vi "New DynamicPersonality.vi"(6 "Pinned":T9={"Attacker"="None", "Striker"="None", "Defender"="None", "Goalie"="None"}, 9 "Maior prioridade de \natacante é o mais\nproximo da bola?":bool, 10 "our_goalie_id":dbl, 11 "input cluster":T1) -> (2 "output cluster":T1)   [LabVIEW 2016]
uses:
  Util/Select Auto None or Robot.ctl
  Core/AI Input.ctl
  Core/AI Robot.ctl
  Intel/Functions Enum.ctl
  Core/AI Ball.ctl
  Core/Field Size.ctl
  Core/AI Judge.ctl
  Intel/Command Enum.ctl
panel:
  out "Strk\nPinned?":bool
  out "Attck\nPinned?":bool
  in  "Ids validos":u32[](array[numeric])=[42, 42, 42, 42, 42, 42, 42]
  in  "Total de Robôs":dbl format="%#_13g"
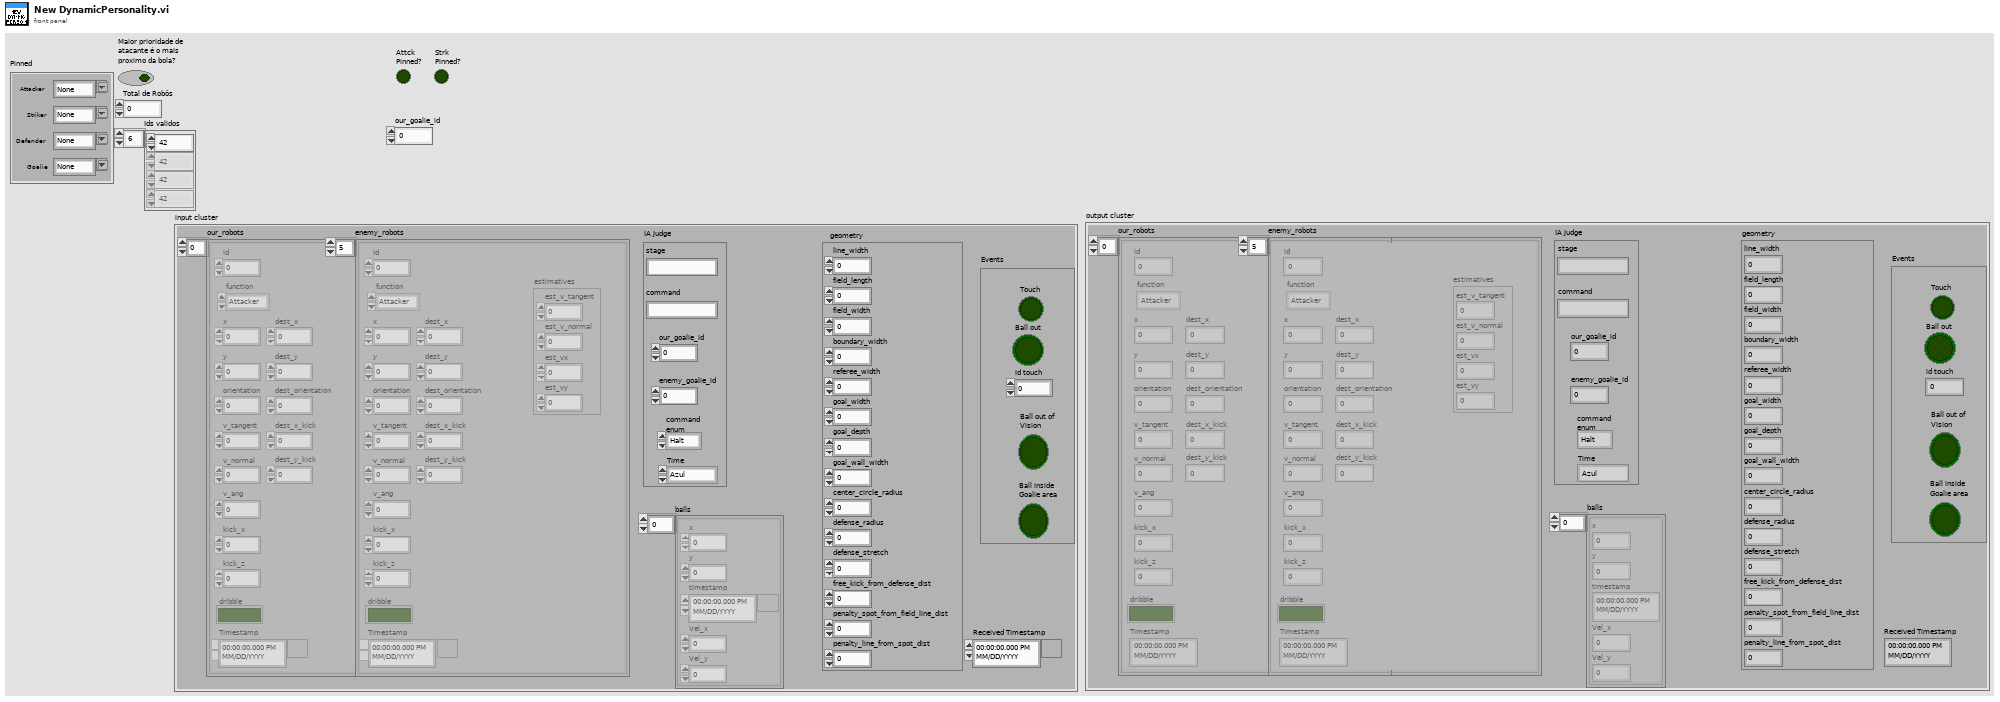
[diagram p1: front panel]
types:
  T1 = typedef "AI Input.ctl" = cluster{"our_robots":T2[], "enemy_robots":T2[], "balls":T4[], "geometry":T5, "IA Judge":T6, "Received Timestamp":timestamp, "Events":cluster{"Touch":bool, "Ball out":bool, "id touch":dbl, "Ball out of \nVision":bool, "Ball inside \nGoalie area":bool}}
  T2 = typedef "AI Robot.ctl" = cluster{"id":u32, "function":T3, "x":dbl, "y":dbl, "orientation":dbl, "v_tangent":dbl, "v_normal":dbl, "v_ang":dbl, "kick_x":dbl, "kick_z":dbl, "dribble":bool, "Timestamp":timestamp, "dest_x":dbl, "dest_y":dbl, "dest_orientation":dbl, "estimatives":cluster{"est_v_tangent":dbl, "est_v_normal":dbl, "est_vx":dbl, "est_vy":dbl}, "dest_x_kick":dbl, "dest_y_kick":dbl}
  T3 = typedef "Functions Enum.ctl" = enum16{"Attacker", "Goalie", "Defender", "Striker", "Goto 0", "Dummy", "ZigZag"}
  T4 = typedef "AI Ball.ctl" = cluster{"x":dbl, "y":dbl, "timestamp":timestamp, "Vel_x":dbl, "Vel_y":dbl}
  T5 = typedef "Field Size.ctl" = cluster{"line_width":u32, "field_length":u32, "field_width":u32, "boundary_width":u32, "referee_width":u32, "goal_width":u32, "goal_depth":u32, "goal_wall_width":u32, "center_circle_radius":u32, "defense_radius":u32, "defense_stretch":u32, "free_kick_from_defense_dist":u32, "penalty_spot_from_field_line_dist":u32, "penalty_line_from_spot_dist":u32}
  T6 = typedef "AI Judge.ctl" = cluster{"stage":string, "command":string, "our_goalie_id":dbl, "enemy_goalie_id":dbl, "command\nenum":T7, "Time":enum16{"Azul", "Amarelo"}}
  T7 = typedef "Command Enum.ctl" = enum16{"Halt", "Stop", "Force Start", "PKA Normal Start", "Prepare Kickoff Ally", "PKE Normal Start", "Prepare Kickoff Enemy", "Prepare Penalty Ally", "PPA Normal Start", "Prepare Penalty Enemy", "PPE Normal Start", "Direct Free Enemy", "Direct Free Ally", "Indirect Free Enemy", "Indirect Free Ally", "Timeout Enemy", "Timeout Ally", "Goal Enemy", "Goal Ally", "Ball Placement Enemy", "Ball Placement Ally", "None"}
  T8 = typedef "Select Auto None or Robot.ctl" = string
  T9 = cluster{"Attacker":T8, "Striker":T8, "Defender":T8, "Goalie":T8}
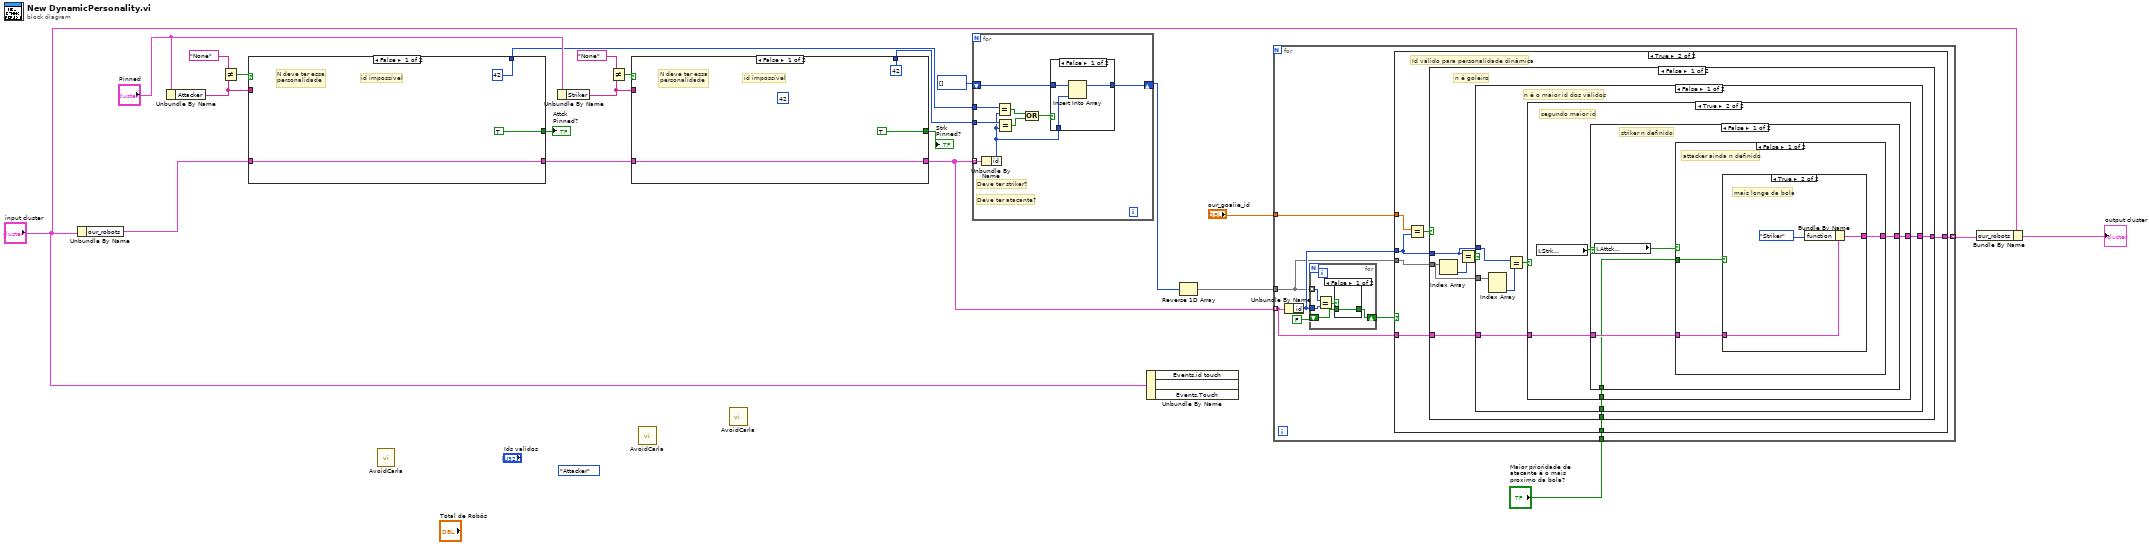
[diagram p0: block diagram]
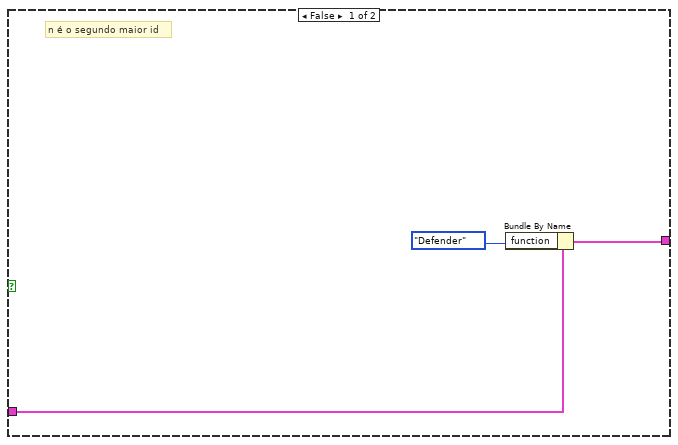
[diagram p3: hidden frame]
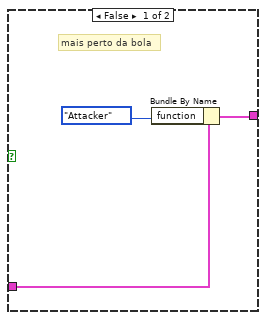
[diagram p4: hidden frame]
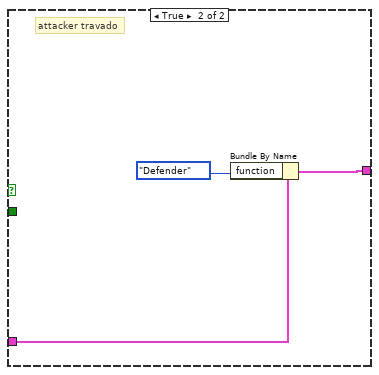
[diagram p5: hidden frame]
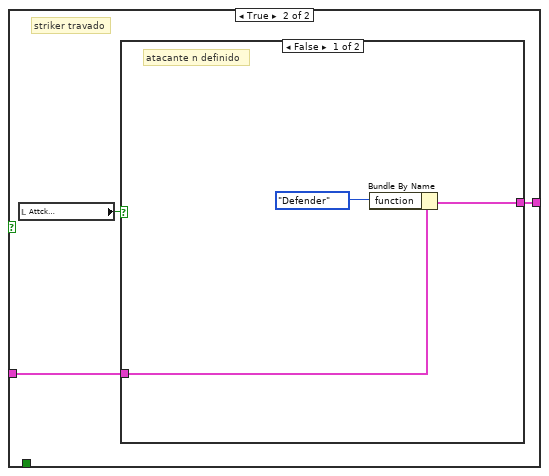
[diagram p6: hidden frame]
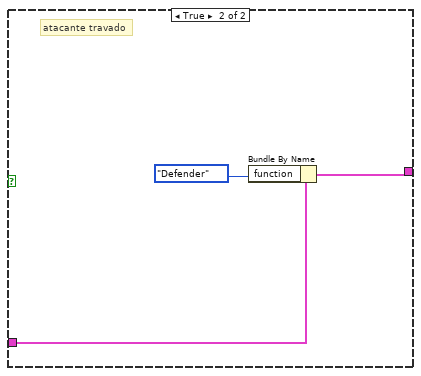
[diagram p7: hidden frame]
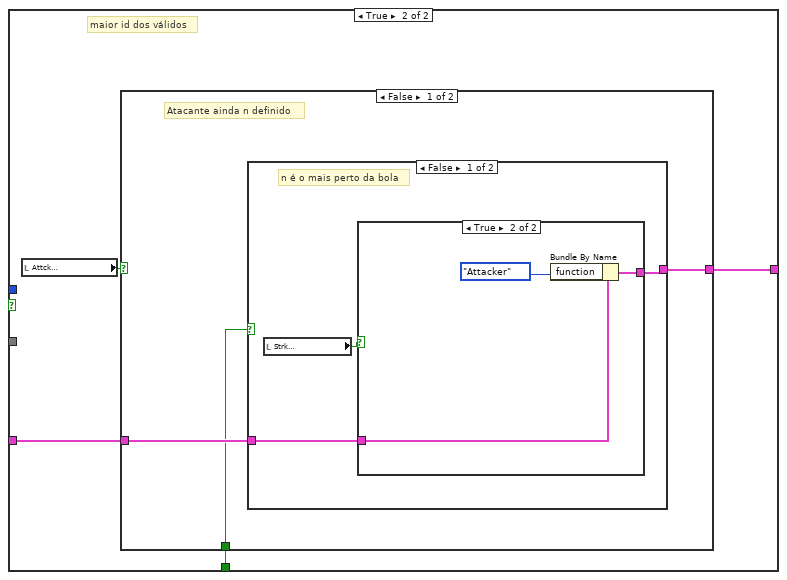
[diagram p8: hidden frame]
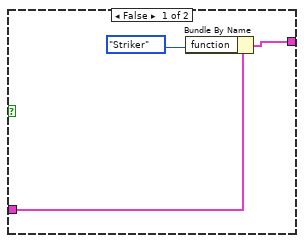
[diagram p9: hidden frame]
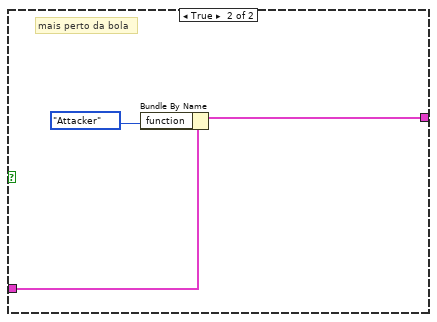
[diagram p10: hidden frame]
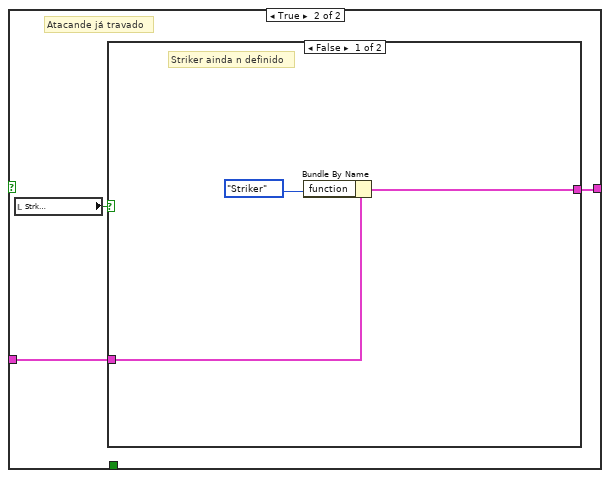
[diagram p11: hidden frame]
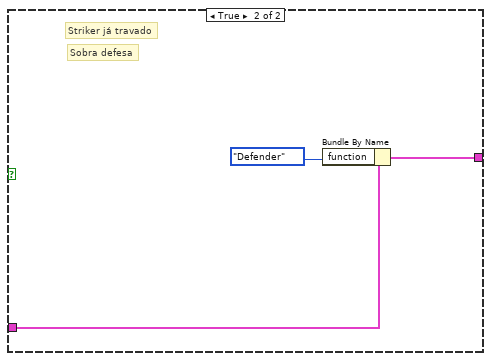
[diagram p12: hidden frame]
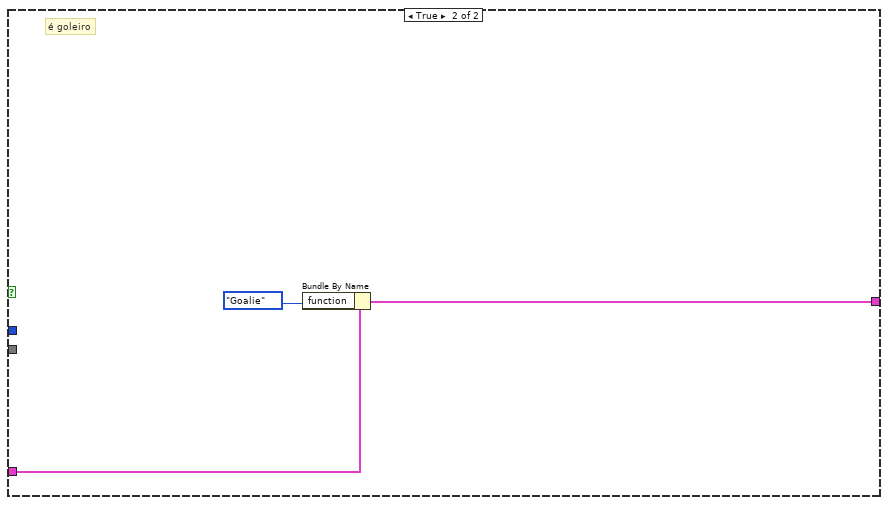
[diagram p13: hidden frame]
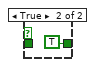
[diagram p14: hidden frame]
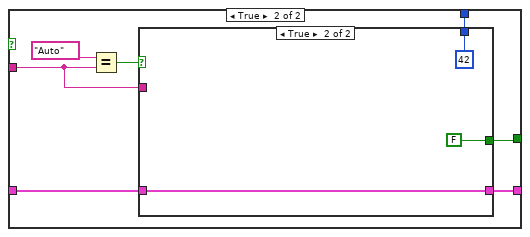
[diagram p16: hidden frame]
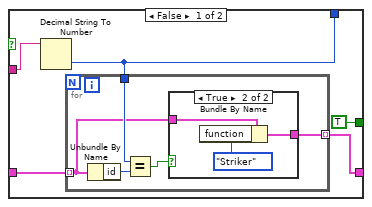
[diagram p17: hidden frame]
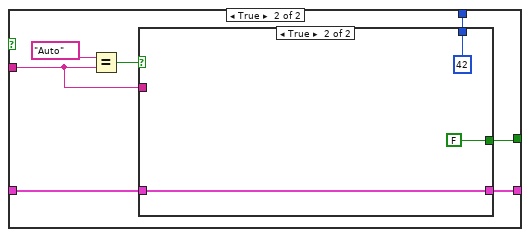
[diagram p19: hidden frame]
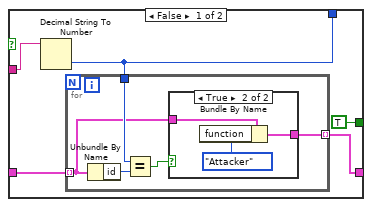
[diagram p20: hidden frame]
diagram:
  (unwired) Functions_Enum."Attacker" ("function")
  n1 = Unbundle By Name("input cluster") -> ("our_robots"=w19:T2[])
  n2 = Unbundle By Name("Pinned") -> ("Attacker"=w20:T8)
  n3 = Not Equal?(x=T8 "None", y=w20) -> (x != y?=w21:bool)
  n4 = case shown="False" w21 {
    tunnel: w20 -> [_ w30]
    tunnel: w19 -> [w25 w29]
    tunnel: [w25 w28] -> w15
    tunnel: [TRUE w27] -> w6
    tunnel: [u32 42 ("Id Maior\nprioridade\natacante") w26] -> w12
    frame False {
      # "id impossível"
      # "N deve ter essa \npersonalidade"
    }
    frame True {
      n5 = Equal?(x=T8 "Auto", y=w30) -> (x = y?=w31:bool)
      n6 = case shown="True" w31 {
        tunnel: w30 -> [w37 _]
        tunnel: w29 -> [w36 w49]
        tunnel: [w35 w49] -> w28
        tunnel: [TRUE FALSE] -> w27
        tunnel: [w33 42] -> w26
        frame False {
          n7 = Decimal String To Number(string=w37) -> (number=w33:i32)  [unwired: 2 in, 1 out]
          n8 = for {
            tunnel: w36 -> [w40] mode=indexing
            tunnel: w33 -> [w41]
            tunnel: [w39] -> w35 mode=indexing
            n9 = Unbundle By Name(w40) -> ("id"=w42:u32)
            n10 = Equal?(x=w41, y=w42) -> (x = y?=w38:bool)
            n11 = case shown="True" w38 {
              tunnel: w40 -> [w43 w46]
              tunnel: [w43 w45] -> w39
              frame False {
              }
              frame True {
                n12 = Bundle By Name(cluster=w46, "function"=Functions_Enum."Attacker") -> (w45:T2)
              }
            }
          }
        }
        frame True {
        }
      }
    }
  }
  "Attck\nPinned?" <- w6
  n13 = call "AvoidCarla.vi"() -> ()  [unwired: 11 in, 1 out]
  n14 = Unbundle By Name("Pinned") -> ("Striker"=w17:T8)
  n15 = Not Equal?(x=T8 "None", y=w17) -> (x != y?=w14:bool)
  n16 = case shown="False" w14 {
    tunnel: w17 -> [_ w57]
    tunnel: w15 -> [w52 w56]
    tunnel: [w52 w55] -> w10
    tunnel: [TRUE w54] -> w5
    tunnel: [42 w53] -> w13
    frame False {
      (unwired) u32 42 ("Id Maior\nprioridade\natacante")
      # "id impossível"
      # "N deve ter essa \npersonalidade"
    }
    frame True {
      n17 = Equal?(x=T8 "Auto", y=w57) -> (x = y?=w58:bool)
      n18 = case shown="True" w58 {
        tunnel: w57 -> [w64 _]
        tunnel: w56 -> [w63 w76]
        tunnel: [w62 w76] -> w55
        tunnel: [TRUE FALSE] -> w54
        tunnel: [w60 42] -> w53
        frame False {
          n19 = Decimal String To Number(string=w64) -> (number=w60:i32)  [unwired: 2 in, 1 out]
          n20 = for {
            tunnel: w63 -> [w67] mode=indexing
            tunnel: w60 -> [w68]
            tunnel: [w66] -> w62 mode=indexing
            n21 = Unbundle By Name(w67) -> ("id"=w69:u32)
            n22 = Equal?(x=w68, y=w69) -> (x = y?=w65:bool)
            n23 = case shown="True" w65 {
              tunnel: w67 -> [w70 w73]
              tunnel: [w70 w72] -> w66
              frame False {
              }
              frame True {
                n24 = Bundle By Name(cluster=w73, "function"=Functions_Enum."Striker") -> (w72:T2)
              }
            }
          }
        }
        frame True {
        }
      }
    }
  }
  "Strk\nPinned?" <- w5
  n25 = call "AvoidCarla.vi"() -> ()  [unwired: 11 in, 1 out]
  n26 = call "AvoidCarla.vi"() -> ()  [unwired: 11 in, 1 out]
  n27 = for {
    tunnel: w10 -> [w85] mode=indexing
    tunnel: w13 -> [w84]
    shift-right: [w79] -> w8
    shift-left: u32[] [] -> [w80]
    tunnel: w12 -> [w83]
    # "Deve ter striker?"
    # "Deve ter atacante?"
    n28 = Unbundle By Name(w85) -> ("id"=w77:u32)
    n29 = Equal?(x=w83, y=w77) -> (x = y?=w82:bool)
    n30 = Equal?(x=w84, y=w77) -> (x = y?=w81:bool)
    n31 = Compound Arithmetic op=OR(w82, w81) -> (w78:bool)
    n32 = case shown="False" w78 {
      tunnel: [w86 w89] -> w79
      tunnel: w80 -> [w88 w89]
      tunnel: w77 -> [w87 _]
      frame False {
        n33 = Insert Into Array(array=w88, new element=w87) -> (w86:u32[])  [unwired: 1 in]
      }
      frame True {
      }
    }
  }
  n34 = Unbundle By Name("input cluster") -> ()  [unwired: 3 out]
  n35 = Reverse 1D Array(array=w8) -> (reversed array=w7:u32[])
  n36 = for {
    tunnel: w10 -> [w94] mode=indexing
    tunnel: w7 -> [w92]
    tunnel: "our_goalie_id" -> [w95]
    tunnel: [w93] -> w4 mode=indexing
    tunnel: "Maior prioridade de \natacante é o mais\nproximo da bola?" -> [w90]
    n37 = Unbundle By Name(w94) -> ("id"=w96:u32)
    n38 = for {
      tunnel: w92 -> [w186] mode=indexing
      tunnel: w96 -> [w187]
      shift-right: [w184] -> w91
      shift-left: FALSE -> [w185]
      n39 = Equal?(x=w186, y=w187) -> (x = y?=w183:bool)
      n40 = case shown="False" w183 {
        tunnel: w185 -> [w188 _]
        tunnel: [w188 TRUE] -> w184
        frame False {
        }
        frame True {
        }
      }
    }
    n41 = case shown="True" w91 {
      tunnel: w96 -> [_ w101]
      tunnel: w95 -> [_ w105]
      tunnel: w94 -> [w98 w103]
      tunnel: [w98 w102] -> w93
      tunnel: w92 -> [_ w100]
      tunnel: w90 -> [_ w99]
      frame False {
        # "Personalidade já definida"
      }
      frame True {
        # "Id válido para personalidade dinâmica"
        n42 = Equal?(x=w105, y=w101) -> (x = y?=w104:bool)
        n43 = case shown="False" w104 {
          tunnel: w103 -> [w109 w181]
          tunnel: [w110 w180] -> w102
          tunnel: w101 -> [w107 _]
          tunnel: w100 -> [w108 _]
          tunnel: w99 -> [w106 _]
          frame False {
            # "n é goleiro"
            n44 = Index Array(array=w108) -> (element=w111:u32)  [unwired: 1 in]
            n45 = Equal?(x=w107, y=w111) -> (x = y?=w112:bool)
            n46 = case shown="False" w112 {
              tunnel: [w116 w154] -> w110
              tunnel: w109 -> [w117 w153]
              tunnel: w108 -> [w118 _]
              tunnel: w107 -> [w115 _]
              tunnel: w106 -> [w113 w152]
              frame False {
                # "n é o maior id dos válidos"
                n47 = Index Array(array=w118) -> (element #2=w114:u32)  [unwired: 2 in, 1 out]
                n48 = Equal?(x=w115, y=w114) -> (x = y?=w119:bool)
                n49 = case shown="True" w119 {
                  tunnel: w117 -> [w120 w125]
                  tunnel: [w121 w124] -> w116
                  tunnel: w113 -> [_ w123]
                  frame False {
                    # "n é o segundo maior id"
                    n50 = Bundle By Name(cluster=w120, "function"=Functions_Enum."Defender") -> (w121:T2)
                  }
                  frame True {
                    # "segundo maior id"
                    n51 = local read "Strk\nPinned?"() -> (w126:bool)
                    n52 = case shown="False" w126 {
                      tunnel: w125 -> [w129 w144]
                      tunnel: [w130 w143] -> w124
                      tunnel: w123 -> [w127 _]
                      frame False {
                        # "striker n definido"
                        n53 = local read "Attck\nPinned?"() -> (w128:bool)
                        n54 = case shown="False" w128 {
                          tunnel: [w133 w141] -> w130
                          tunnel: w129 -> [w132 w140]
                          tunnel: w127 -> [w131 _]
                          frame False {
                            # "attacker ainda n definido"
                            n55 = case shown="True" w131 {
                              tunnel: [w135 w138] -> w133
                              tunnel: w132 -> [w134 w137]
                              frame False {
                                # "mais perto da bola"
                                n56 = Bundle By Name(cluster=w134, "function"=Functions_Enum."Attacker") -> (w135:T2)
                              }
                              frame True {
                                # "mais longe da bola"
                                n57 = Bundle By Name(cluster=w137, "function"=Functions_Enum."Striker") -> (w138:T2)
                              }
                            }
                          }
                          frame True {
                            # "attacker travado"
                            n58 = Bundle By Name(cluster=w140, "function"=Functions_Enum."Defender") -> (w141:T2)
                          }
                        }
                      }
                      frame True {
                        # "striker travado"
                        n59 = local read "Attck\nPinned?"() -> (w145:bool)
                        n60 = case shown="False" w145 {
                          tunnel: w144 -> [w146 w149]
                          tunnel: [w147 w150] -> w143
                          frame False {
                            # "atacante n definido"
                            n61 = Bundle By Name(cluster=w146, "function"=Functions_Enum."Defender") -> (w147:T2)
                          }
                          frame True {
                            # "atacante travado"
                            n62 = Bundle By Name(cluster=w149, "function"=Functions_Enum."Defender") -> (w150:T2)
                          }
                        }
                      }
                    }
                  }
                }
              }
              frame True {
                # "maior id dos válidos"
                n63 = local read "Attck\nPinned?"() -> (w155:bool)
                n64 = case shown="False" w155 {
                  tunnel: [w158 w172] -> w154
                  tunnel: w153 -> [w157 w171]
                  tunnel: w152 -> [w156 _]
                  frame False {
                    # "Atacante ainda n definido"
                    n65 = case shown="False" w156 {
                      tunnel: [w161 w169] -> w158
                      tunnel: w157 -> [w160 w168]
                      frame False {
                        # "n é o mais perto da bola"
                        n66 = local read "Strk\nPinned?"() -> (w159:bool)
                        n67 = case shown="True" w159 {
                          tunnel: [w163 w166] -> w161
                          tunnel: w160 -> [w162 w165]
                          frame False {
                            n68 = Bundle By Name(cluster=w162, "function"=Functions_Enum."Striker") -> (w163:T2)
                          }
                          frame True {
                            n69 = Bundle By Name(cluster=w165, "function"=Functions_Enum."Attacker") -> (w166:T2)
                          }
                        }
                      }
                      frame True {
                        # "mais perto da bola"
                        n70 = Bundle By Name(cluster=w168, "function"=Functions_Enum."Attacker") -> (w169:T2)
                      }
                    }
                  }
                  frame True {
                    # "Atacande já travado"
                    n71 = local read "Strk\nPinned?"() -> (w173:bool)
                    n72 = case shown="False" w173 {
                      tunnel: [w175 w178] -> w172
                      tunnel: w171 -> [w174 w177]
                      frame False {
                        # "Striker ainda n definido"
                        n73 = Bundle By Name(cluster=w174, "function"=Functions_Enum."Striker") -> (w175:T2)
                      }
                      frame True {
                        # "Sobra defesa"
                        # "Striker já travado"
                        n74 = Bundle By Name(cluster=w177, "function"=Functions_Enum."Defender") -> (w178:T2)
                      }
                    }
                  }
                }
              }
            }
          }
          frame True {
            # "é goleiro"
            n75 = Bundle By Name(cluster=w181, "function"=Functions_Enum."Goalie") -> (w180:T2)
          }
        }
      }
    }
  }
  n76 = Bundle By Name(cluster="input cluster", "our_robots"=w4) -> (→"output cluster":T1)
